vi "Check License Form Data.vi"(11 "License Form":T1) -> (2 "Warning":string, 3 "Data Valid (F)":bool)   [LabVIEW 2022 SP3]
uses:
  Controls/License Request Form.ctl
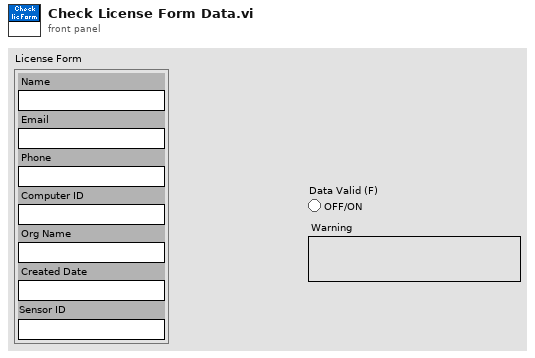
[diagram p1: front panel]
types:
  T1 = typedef "License Request Form.ctl" = cluster{"Name":string, "Email":string, "Phone":string, "Computer ID":string, "Org Name":string, "Created Date":string, "Sensor ID":string}
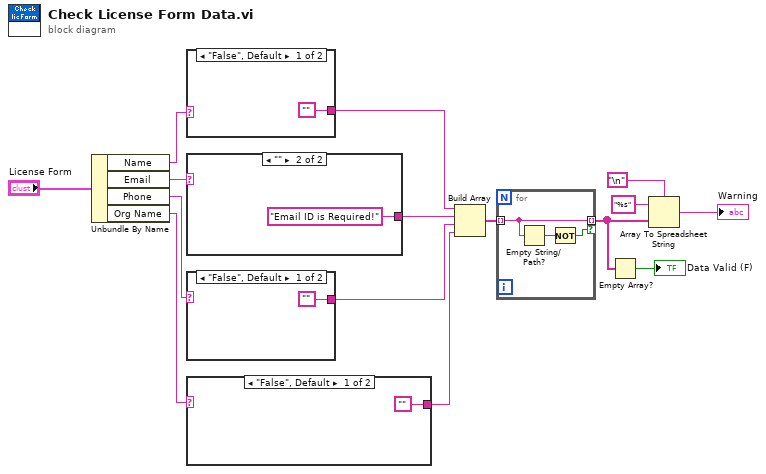
[diagram p0: block diagram]
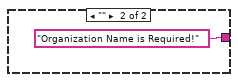
[diagram p2: hidden frame]
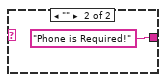
[diagram p3: hidden frame]
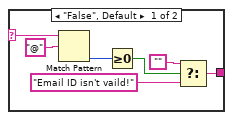
[diagram p4: hidden frame]
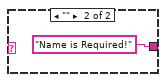
[diagram p5: hidden frame]
diagram:
  n1 = Unbundle By Name("License Form") -> ("Name"=w14:string, "Email"=w13:string, "Phone"=w12:string, "Org Name"=w11:string)
  n2 = case shown="\"False\", Default" w14 {
    tunnel: ["" ("t") "Name is Required!"] -> w10
    frame "False", Default {
    }
    frame "" {
    }
  }
  n3 = case shown="\"\"" w13 {
    selector: w13 -> [w24 _]
    tunnel: [w18 "Email ID is Required!"] -> w9
    frame "False", Default {
      n4 = Match Pattern(string=w24, regular expression="@") -> (offset past match=w22:i32)  [unwired: 1 in, 3 out]
      n5 = Greater Or Equal To 0?(x=w22) -> (x >= 0?=w21:bool)
      n6 = Select(t="", s=w21, f="Email ID isn't vaild!") -> (s? t:f=w18:string)
    }
    frame "" {
    }
  }
  n7 = case shown="\"False\", Default" w12 {
    tunnel: ["" ("t") "Phone is Required!"] -> w8
    frame "False", Default {
    }
    frame "" {
    }
  }
  n8 = case shown="\"False\", Default" w11 {
    tunnel: ["" ("t") "Organization Name is Required!"] -> w7
    frame "False", Default {
    }
    frame "" {
    }
  }
  n9 = Build Array(w10, w9, w8, w7) -> (w6:string[])
  n10 = for {
    tunnel: w6 -> [w32] mode=indexing
    tunnel: [w32] -> w2 mode=indexing if=w30
    n11 = Empty String/Path?(string/path=w32) -> (empty?=w31:bool)
    n12 = Not(x=w31) -> (.not. x?=w30:bool)
  }
  n13 = Empty Array?(array=w2) -> (empty?=→"Data Valid (F)":bool)
  n14 = Array To Spreadsheet String(delimiter (Tab)="\n", array=w2, 3:"%s" ("format string")) -> (spreadsheet string=→"Warning":string)
